vi "DWF MSO Configure Immediate Trigger.vi"(0 "Instrument Handle In":u32, 11 "Error In":errorcluster caption="Error In (no error)") -> (4 "Instrument Handle Out":u32, 15 "Error Out":errorcluster)   [LabVIEW 2015, in "DigilentWF.lvlib"]
doc: "Configures a trigger to immediately activate on the specified channels after the pretrigger time has expired."
uses:
  <vilib>/DigilentWF/DigilentWF.lvlib
  dwf.dll
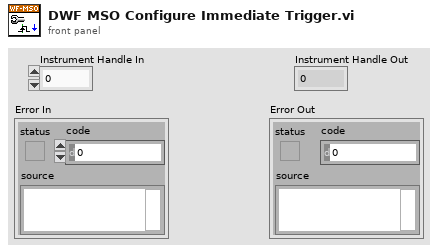
[diagram p1: front panel]
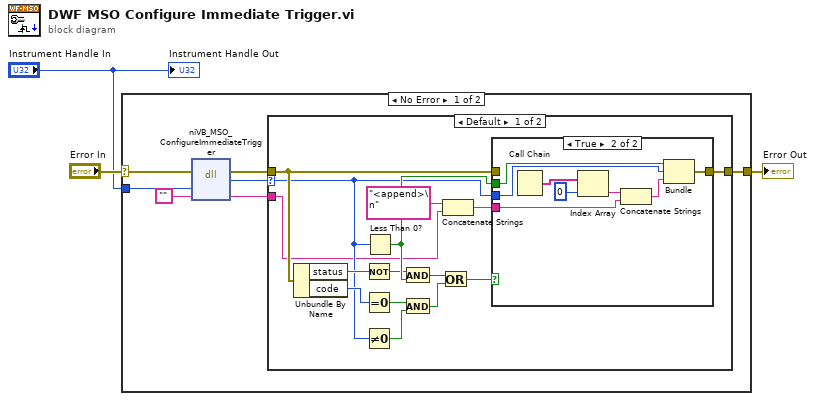
[diagram p0: block diagram]
diagram:
  n1 = case "outter_case" shown="No Error" "Error In" {
    selector: "Error In" -> [w10 w36]
    tunnel: [w7 w36] -> w2
    tunnel: "Instrument Handle In" -> [w6 _]
    frame No Error {
      n2 = dll-call lib="dwf.*" fn="niVB_MSO_ConfigureImmediateTrigger"(error in=w10, "InstrumentHandle"=w6, "szError"="") -> (error out=w9:errorcluster, "return type"=w8:i32, "szError"=w4:string)  [unwired: 3 in, 1 out]
      n3 = case "inner_case" shown="Default" w8 {
        selector: w8 -> [w15 _]
        tunnel: w9 -> [w16 w35]
        tunnel: [w12 w35] -> w7
        tunnel: w4 -> [w11 _]
        frame Default {
          n4 = Unbundle By Name(w16) -> ("status"=w20:bool, "code"=w24:i32)
          n5 = Not(x=w20) -> (.not. x?=w23:bool)
          n6 = Equal To 0?(x=w24) -> (x = 0?=w19:bool)
          n7 = Not Equal To 0?(x=w15) -> (x != 0?=w22:bool)
          n8 = Less Than 0?(x=w15) -> (x < 0?=w25:bool)
          n9 = And(x=w23, y=w25) -> (x .and. y?=w21:bool)
          n10 = And(x=w19, y=w22) -> (x .and. y?=w18:bool)
          n11 = Or(x=w21, y=w18) -> (x .or. y?=w17:bool)
          n12 = Concatenate Strings("<append>\n" ("string"), w11) -> (w14:string)
          n13 = case shown="True" w17 {
            tunnel: [w26 w33] -> w12
            tunnel: w15 -> [_ w32]
            tunnel: w25 -> [_ w31]
            tunnel: w16 -> [w26 _]
            tunnel: w14 -> [_ w27]
            frame False {
            }
            frame True {
              n14 = Call Chain() -> (call chain=w30:string[])
              n15 = Index Array(array=w30, index=0) -> (element=w29:string)
              n16 = Concatenate Strings(w29, w27) -> (w34:string)
              n17 = Bundle(w31, "return type"=w32, w34) -> (w33:cluster{bool, "return type":i32, string})  [unwired: 1 out]
            }
          }
        }
        frame 0 {
        }
      }
    }
    frame Error {
    }
  }
  "Error Out" <- w2
  "Instrument Handle Out" <- "Instrument Handle In"
